vi "String Subset.vi"(3 "Offset past End":i32=-1, 4 "Start offset":i32, 5 "JSON":string) -> (1 "substring":string)   [LabVIEW 2021, in "json.facade.lvlib"]
doc: "String subset between two offsets."
uses:
  json.facade.lvlib
  jsontext/JSONtext.lvlib
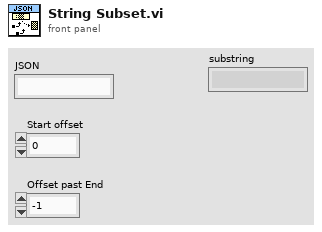
[diagram p1: front panel]
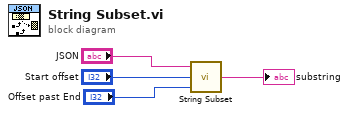
[diagram p0: block diagram]
diagram:
  n1 = call "String Subset.vi"("Offset past End"="Offset past End", "Start offset"="Start offset", "JSON"="JSON") -> ("substring"=→"substring":string)  [unwired: 2 in]
